vi "SUMMITEK Create Registry Key.vi"(5 "machine (local)":string, 6 "class":string, 7 "options":T2(ring), 8 "error in (no error)":errorcluster, 9 "security access mask (KEY_READ | KEY_WRITE)":T4=enum."KEY_READ | KEY_WRITE", 10 "subkey":string, 11 "root key (HKEY_LOCAL_MACHINE)":T5=enum."HKEY_LOCAL_MACHINE") -> (0 "error out":errorcluster, 2 "action taken":T1(ring)=enum."REG_CREATED_NEW_KEY", 3 "refnum out":T3)   [LabVIEW 2011]
doc: "Creates a key in the Windows Registry or opens it, if it already exists."
uses:
  <vilib>/registry/registry.llb/Registry RtKey.ctl
  <vilib>/registry/registry.llb/Registry SAM.ctl
  <vilib>/registry/registry.llb/Registry refnum.ctl
  Advapi32.dll
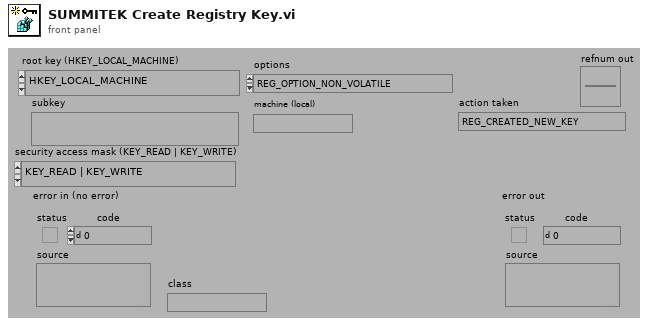
[diagram p1: front panel]
types:
  T1 = enum32{"Unknown", "REG_CREATED_NEW_KEY", "REG_OPENED_EXISTING_KEY"}
  T2 = enum32{"REG_OPTION_NON_VOLATILE", "REG_OPTION_VOLATILE", "REG_OPTION_BACKUP_RESTORE"}
  T3 = typedef "Registry refnum.ctl" = refnum<k1>
  T4 = typedef "Registry SAM.ctl" = enum32{"KEY_QUERY_VALUE", "KEY_SET_VALUE", "KEY_CREATE_SUB_KEY", "KEY_ENUMERATE_SUB_KEYS", "KEY_NOTIFY", "KEY_CREATE_LINK", "KEY_READ", "KEY_WRITE", "KEY_ALL_ACCESS", "KEY_READ | KEY_WRITE"}
  T5 = typedef "Registry RtKey.ctl" = enum32{"HKEY_CLASSES_ROOT", "HKEY_CURRENT_USER", "HKEY_LOCAL_MACHINE", "HKEY_USERS", "HKEY_PERFORMANCE_DATA", "HKEY_CURRENT_CONFIG", "HKEY_DYN_DATA"}
  T6 = enum16{"store handles", "dispose handles", "get handles"}
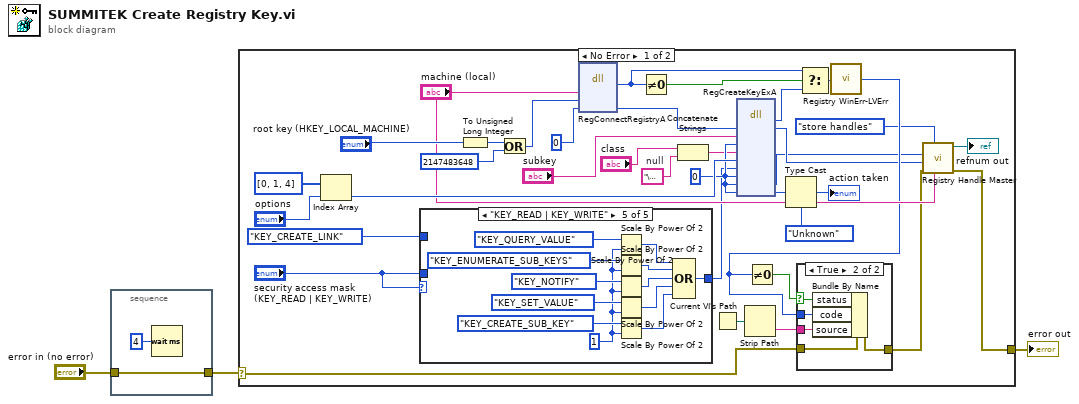
[diagram p0: block diagram]
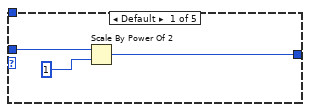
[diagram p3: hidden frame]
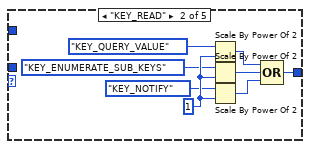
[diagram p4: hidden frame]
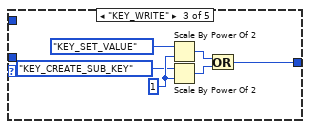
[diagram p5: hidden frame]
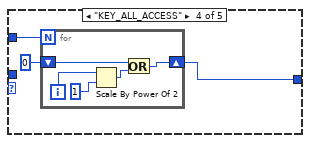
[diagram p6: hidden frame]
diagram:
  n1 = stacked-sequence {
    tunnel: "error in (no error)" -> [w4]
    tunnel: [w4] -> w1
    frame #0 {
      n2 = Wait (ms)(milliseconds to wait=u32 4) -> ()  [unwired: 1 out]
    }
  }
  n3 = case shown="No Error" w1 {
    selector: w1 -> [w10 w85]
    tunnel: [w9 w85] -> w3
    frame No Error {
      w17 = "\u0000"  # null
      w30 = u32 0 ("lpSecurityAttributes[NULL]")
      n4 = Index Array(array=u32[] [0, 1, 4], index="options") -> (element=w32:u32)
      n5 = case shown="\"KEY_READ | KEY_WRITE\"" "security access mask (KEY_READ | KEY_WRITE)" {
        tunnel: [w50 w58 w59 w65 w75] -> w20
        tunnel: "security access mask (KEY_READ | KEY_WRITE)" -> [w48 _ _ _ _]
        tunnel: Registry_SAM."KEY_CREATE_LINK" ("security access mask (KEY_READ | KEY_WRITE)") -> [_ _ _ w66 _]
        frame Default {
          n6 = Scale By Power Of 2(n=w48, x=u32 1) -> (x*2^n=w50:u32)
        }
        frame "KEY_READ" {
          w57 = u32 1
          n7 = Scale By Power Of 2(n=Registry_SAM."KEY_QUERY_VALUE" ("security access mask (KEY_READ | KEY_WRITE)"), x=w57) -> (x*2^n=w54:u32)
          n8 = Scale By Power Of 2(n=Registry_SAM."KEY_ENUMERATE_SUB_KEYS" ("security access mask (KEY_READ | KEY_WRITE)"), x=w57) -> (x*2^n=w56:u32)
          n9 = Scale By Power Of 2(n=Registry_SAM."KEY_NOTIFY" ("security access mask (KEY_READ | KEY_WRITE)"), x=w57) -> (x*2^n=w55:u32)
          n10 = Compound Arithmetic op=OR(w54, w56, w55) -> (w58:u32)
        }
        frame "KEY_WRITE" {
          w62 = u32 1
          n11 = Scale By Power Of 2(n=Registry_SAM."KEY_SET_VALUE" ("security access mask (KEY_READ | KEY_WRITE)"), x=w62) -> (x*2^n=w63:u32)
          n12 = Scale By Power Of 2(n=Registry_SAM."KEY_CREATE_SUB_KEY" ("security access mask (KEY_READ | KEY_WRITE)"), x=w62) -> (x*2^n=w64:u32)
          n13 = Or(x=w63, y=w64) -> (x .or. y?=w59:u32)
        }
        frame "KEY_ALL_ACCESS" {
          n14 = for {
            N: w66 -> [_]
            shift-right: [w69] -> w65
            shift-left: u32 0 -> [w70]
            i -> [w71]
            n15 = Scale By Power Of 2(n=w71, x=u32 1) -> (x*2^n=w68:u32)
            n16 = Or(x=w70, y=w68) -> (x .or. y?=w69:u32)
          }
        }
        frame "KEY_READ | KEY_WRITE" {
          w76 = u32 1
          n17 = Scale By Power Of 2(n=Registry_SAM."KEY_QUERY_VALUE" ("security access mask (KEY_READ | KEY_WRITE)"), x=w76) -> (x*2^n=w82:u32)
          n18 = Scale By Power Of 2(n=Registry_SAM."KEY_ENUMERATE_SUB_KEYS" ("security access mask (KEY_READ | KEY_WRITE)"), x=w76) -> (x*2^n=w84:u32)
          n19 = Scale By Power Of 2(n=Registry_SAM."KEY_NOTIFY" ("security access mask (KEY_READ | KEY_WRITE)"), x=w76) -> (x*2^n=w83:u32)
          n20 = Scale By Power Of 2(n=Registry_SAM."KEY_SET_VALUE" ("security access mask (KEY_READ | KEY_WRITE)"), x=w76) -> (x*2^n=w74:u32)
          n21 = Scale By Power Of 2(n=Registry_SAM."KEY_CREATE_SUB_KEY" ("security access mask (KEY_READ | KEY_WRITE)"), x=w76) -> (x*2^n=w73:u32)
          n22 = Compound Arithmetic op=OR(w82, w84, w83, w74, w73) -> (w75:u32)
        }
      }
      n23 = To Unsigned Long Integer(number="root key (HKEY_LOCAL_MACHINE)") -> (unsigned 32bit integer=w41:u32)
      n24 = Or(x=w41, y=u32 2147483648) -> (x .or. y?=w28:u32)
      n25 = dll-call lib="Advapi32.dll" fn="RegConnectRegistryA"("lpMachineName"="machine (local)", "hKey"=w28, "phkResult"=u32 0) -> (w24:i32, "phkResult"=w27:u32)  [unwired: 4 in, 3 out]
      n26 = Not Equal To 0?(x=w24) -> (x != 0?=w25:bool)
      n27 = Concatenate Strings("class", w17) -> (w18:string)
      n28 = Current VI's Path() -> (path=w36:path)
      n29 = dll-call lib="Advapi32.dll" fn="RegCreateKeyExA"("hKey"=w27, "lpSubKey"="subkey", "dwReserved"=w30, "lpClass"=w18, "dwOptions"=w32, "samDesired"=w20, "lpSecurityAttributes[NULL]"=w30, "phkResult"=w30, "lpdwDisposition"=w30) -> (w23:i32, "hKey"=w8:u32, "phkResult"=w7:u32, "lpdwDisposition"=w31:u32)  [unwired: 9 in, 2 out]
      n30 = Strip Path(path=w36) -> (name=w37:string)  [unwired: 1 out]
      n31 = Type Cast(type=T1."Unknown" ("action taken"), x=w31) -> (*(type *) &x=→"action taken":T1)
      n32 = Select(t=w24, s=w25, f=w23) -> (s? t:f=w22:i32)
      n33 = call <vilib>:"Registry WinErr-LVErr.vi"("Windows error"=w22) -> ("LabVIEW error"=w16:i32)  [unwired: 4 out]
      n34 = Not Equal To 0?(x=w16) -> (x != 0?=w15:bool)
      n35 = case shown="True" w15 {
        selector: w15 -> [_ w43]
        tunnel: w37 -> [_ w47]
        tunnel: [w42 w46] -> w6
        tunnel: w16 -> [_ w45]
        tunnel: w10 -> [w42 w44]
        frame False {
        }
        frame True {
          n36 = Bundle By Name(cluster=w44, "status"=w43, "code"=w45, "source"=w47) -> (w46:errorcluster)
        }
      }
      n37 = call <vilib>:"Registry Handle Master.vi"("machine"="machine (local)", "action (get handles)"=T6."store handles", "error in (no error)"=w6, "remote key handle"=w8, "key handle"=w7) -> ("error out"=w9:errorcluster, "refnum out"=→"refnum out":T3)  [unwired: 1 in, 4 out]
    }
    frame Error {
    }
  }
  "error out" <- w3
